vi "specu1a 1.0.0 Param Enum to Param Cluster.vi"(1 "Parameters":T1={"Integration time"=10000, "Gain"=enum."No Function", "TriggerEdge"=enum."No Function", "Trigger Mode"=enum."Asynchronous", "Reserved"=0}) -> (0 "Cluster in":T4)   [LabVIEW 2019]
uses:
  Controls/specu1a 1.0.0 Parameters.ctl
  Controls/specu1a 1.0.0 Trigger Edge.ctl
  Controls/specu1a 1.0.0 Trigger Mode.ctl
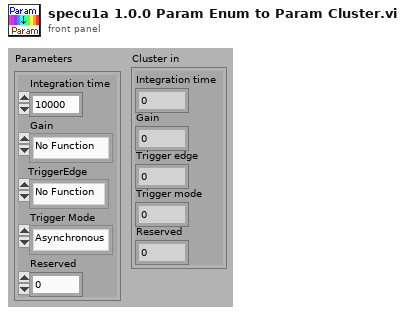
[diagram p1: front panel]
types:
  T1 = typedef "specu1a 1.0.0 Parameters.ctl" = cluster{"Integration time":u32, "Gain":enum16{"Low", "High", "No Function"}, "TriggerEdge":T2, "Trigger Mode":T3, "Reserved":u8}
  T2 = typedef "specu1a 1.0.0 Trigger Edge.ctl" = enum16{"Rising", "Falling", "No Function"}
  T3 = typedef "specu1a 1.0.0 Trigger Mode.ctl" = enum16{"Internal", "Asynchronous", "Synchronous"}
  T4 = cluster{"Integration time":u32, "Gain":u8, "Trigger edge":u8, "Trigger mode":u8, "Reserved":u8}
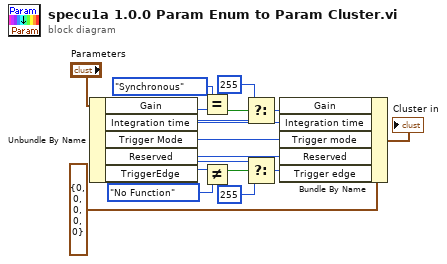
[diagram p0: block diagram]
diagram:
  n1 = Unbundle By Name("Parameters") -> ("Gain"=w10:enum16{"Low", "High", "No Function"}, "Integration time"=w14:u32, "Trigger Mode"=w16:T3, "Reserved"=w15:u8, "TriggerEdge"=w3:T2)
  n2 = Equal?(x=specu1a_1.0.0_Trigger_Mode."Synchronous" ("Gain"), y=w10) -> (x = y?=w9:bool)
  n3 = Not Equal?(x=w3, y=specu1a_1.0.0_Trigger_Edge."No Function" ("TriggerEdge")) -> (x != y?=w2:bool)
  n4 = Select(t=255, s=w9, f=w10) -> (s? t:f=w7:i32)
  n5 = Select(t=w3, s=w2, f=255) -> (s? t:f=w4:i32)
  n6 = Bundle By Name(cluster=T4 {"Integration time"=0, "Gain"=0, "Trigger edge"=0, "Trigger mode"=0, "Reserved"=0} ("Cluster in"), "Gain"=w7, "Integration time"=w14, "Trigger mode"=w16, "Reserved"=w15, "Trigger edge"=w4) -> (→"Cluster in":T4)
